vi "Ultrasonic Plot V2015.vi"(0 "Front L/R":cluster{i32, i32}, 4 "Limiter":i16=60, 5 "Y/X/Ang":cluster{"Y":i32, "X":i32, "Ring 2":T1} {"Ring 2" items=["0", "45", "90", "135", "180", "225", "270", "315"]}, 6 "error in (no error)":errorcluster, 7 "map reference in":refnum<data-value>) -> (1 "Runmap":bool, 2 "error out":errorcluster, 3 "map reference out":refnum<data-value>)   [LabVIEW 2014]
uses:
  <vilib>/robotics/Navigation/shared/WorldMap/OccupancyGridWorldMap/NI_Robotics_OccupancyGridWorldMap.lvclass
  Controls/Direction enum.ctl
panel:
  out "s? t:f":i32
  out "Angle":T1 items=["0", "45", "90", "135", "180", "225", "270", "315"]
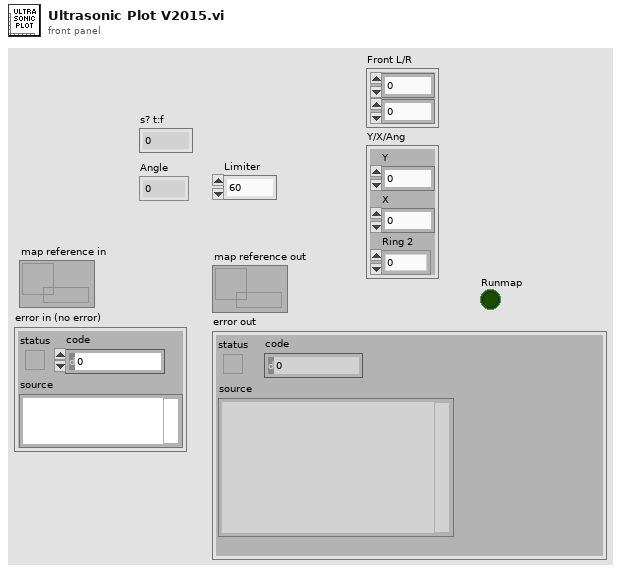
[diagram p1: front panel]
types:
  T1 = typedef "Direction enum.ctl" = u16
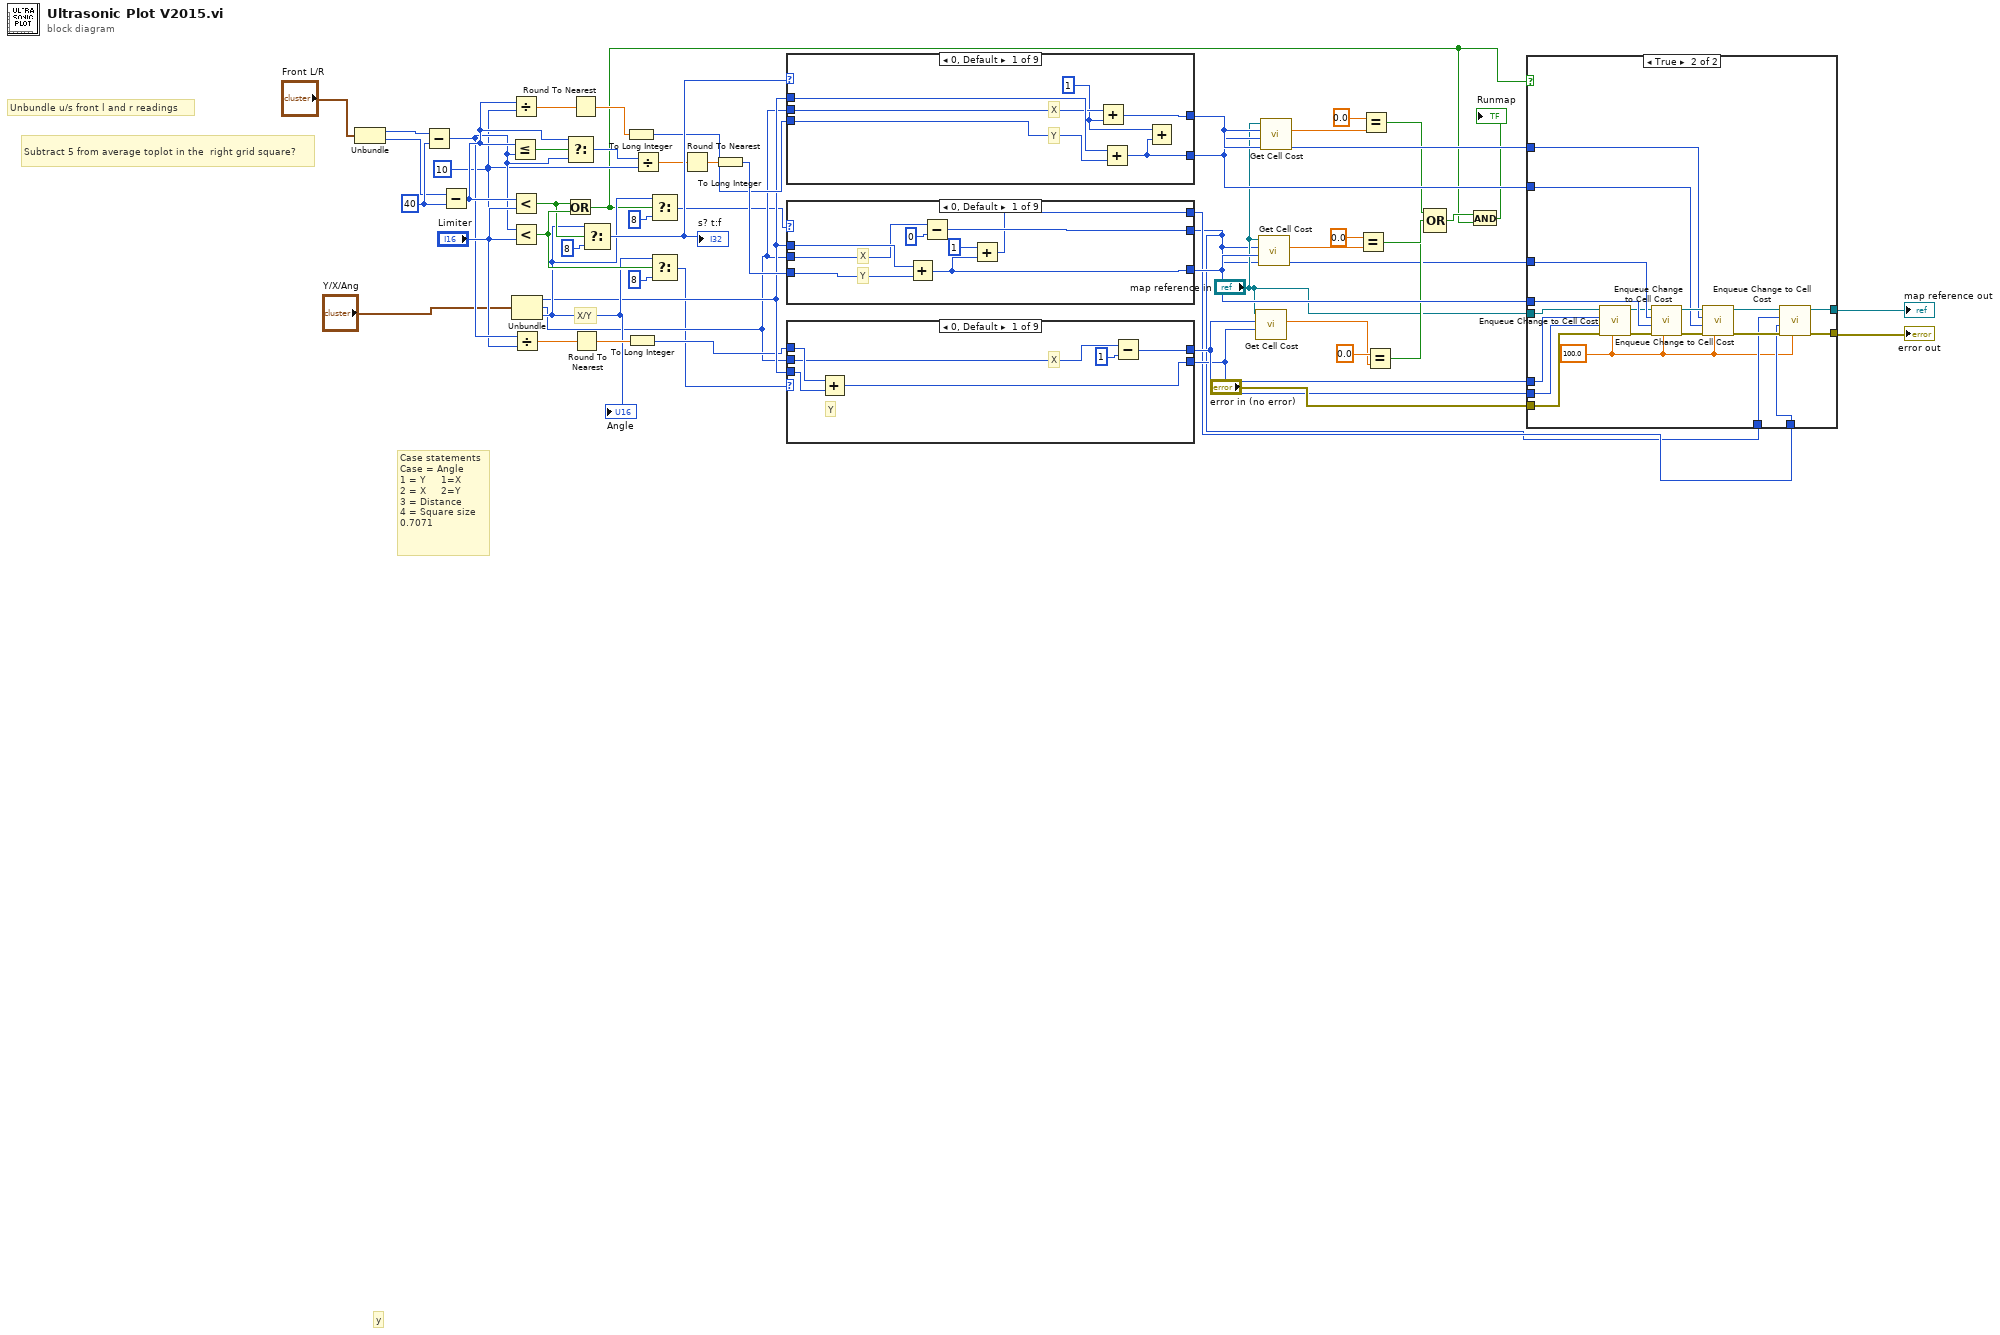
[diagram p0: block diagram]
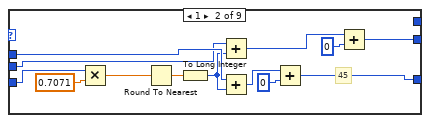
[diagram p2: hidden frame]
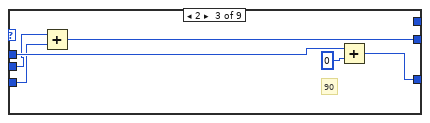
[diagram p3: hidden frame]
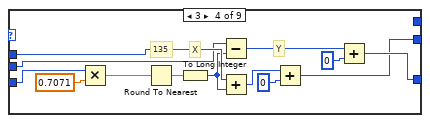
[diagram p4: hidden frame]
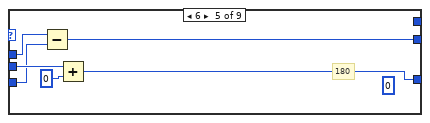
[diagram p5: hidden frame]
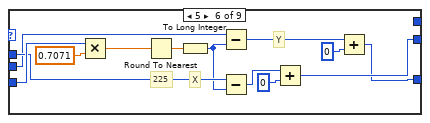
[diagram p6: hidden frame]
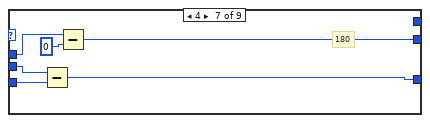
[diagram p7: hidden frame]
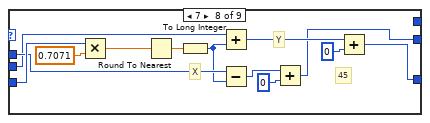
[diagram p8: hidden frame]
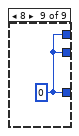
[diagram p9: hidden frame]
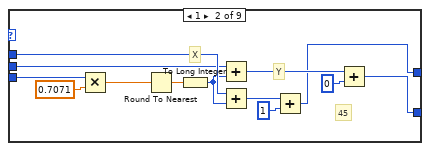
[diagram p10: hidden frame]
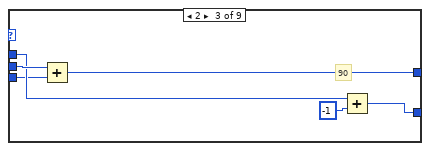
[diagram p11: hidden frame]
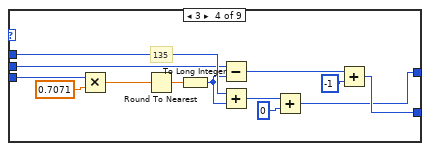
[diagram p12: hidden frame]
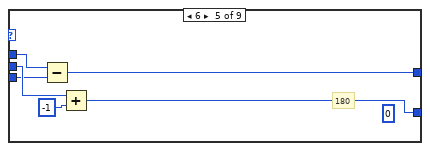
[diagram p13: hidden frame]
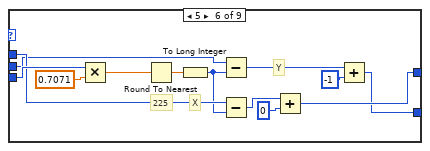
[diagram p14: hidden frame]
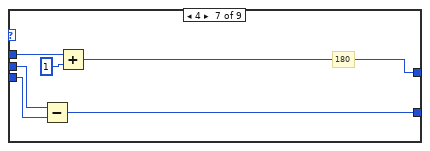
[diagram p15: hidden frame]
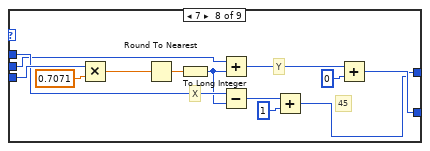
[diagram p16: hidden frame]
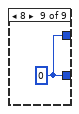
[diagram p17: hidden frame]
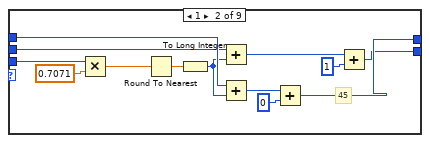
[diagram p18: hidden frame]
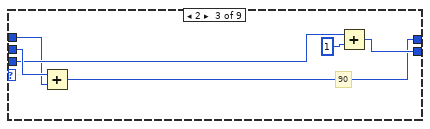
[diagram p19: hidden frame]
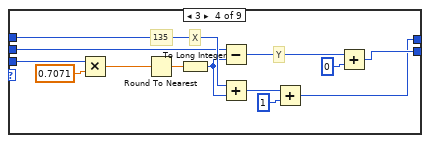
[diagram p20: hidden frame]
diagram:
  w37 = 40
  w33 = 10
  # "Subtract 5 from average toplot in the  right grid square?"
  # "Unbundle u/s front l and r readings"
  # "Case statements \nCase = Angle\n1 = Y     1=X\n2 = X     2=Y\n3 = Distance\n4 = Square size \n0.7071"
  # "y"
  # "X/Y"
  n1 = Unbundle("Front L/R") -> (w31:i32, w30:i32)
  n2 = Subtract(x=w31, y=w37) -> (x-y=w34:i32)
  n3 = Subtract(x=w30, y=w37) -> (x-y=w36:i32)
  n4 = Less Or Equal?(x=w36, y=w34) -> (x <= y?=w51:bool)
  n5 = Divide(x=w36, y=w33) -> (x/y=w45:dbl)
  n6 = Less?(x=w36, y="Limiter") -> (x < y?=w48:bool)
  n7 = Less?(x=w34, y="Limiter") -> (x < y?=w49:bool)
  n8 = Unbundle("Y/X/Ang") -> ("Y"=w7:i32, "X"=w5:i32, "Ring 2"=w27:T1)
  "Angle" <- w27
  n9 = Divide(x=w34, y=w33) -> (x/y=w35:dbl)
  n10 = Select(t=w36, s=w51, f=w34) -> (s? t:f=w42:i32)
  n11 = Or(x=w48, y=w49) -> (x .or. y?=w11:bool)
  n12 = Round To Nearest(number=w45) -> (nearest integer value=w46:dbl)
  n13 = Round To Nearest(number=w35) -> (nearest integer value=w32:dbl)
  n14 = Select(t=w27, s=w48, f=8) -> (s? t:f=w50:i32)
  "s? t:f" <- w50
  n15 = To Long Integer(number=w46) -> (32bit integer=w8:i32)
  n16 = To Long Integer(number=w32) -> (32bit integer=w6:i32)
  n17 = Divide(x=w42, y=w33) -> (x/y=w43:dbl)
  n18 = Select(t=w27, s=w11, f=8) -> (s? t:f=w4:i32)
  n19 = Select(t=w27, s=w49, f=8) -> (s? t:f=w1:i32)
  n20 = Round To Nearest(number=w43) -> (nearest integer value=w44:dbl)
  n21 = To Long Integer(number=w44) -> (32bit integer=w41:i32)
  n22 = case shown="0, Default" w50 {
    tunnel: w5 -> [w59 w68 w78 w87 w96 w106 w113 w125 _]
    tunnel: w7 -> [w60 w71 w77 w90 w97 w109 w116 w128 _]
    tunnel: w8 -> [w55 w73 w76 w92 w93 w111 w112 w130 _]
    tunnel: [w58 w61 w75 w80 w95 w100 w115 w118 w131] -> w26
    tunnel: [w56 w62 w74 w81 w94 w99 w114 w119 w131] -> w25
    frame 0, Default {
      w57 = 1
      # "Y"
      # "X"
      n23 = Add(x=w59, y=w57) -> (x+y=w58:i32)
      n24 = Add(x=w60, y=w55) -> (x+y=w56:i32)
      n25 = Add(x=w57, y=w56) -> ()  [unwired: 1 out]
    }
    frame 1 {
      # "Y"
      # "X"
      # "45"
      n26 = Multiply(x=w73, y=0.7071) -> (x*y=w63:dbl)
      n27 = Round To Nearest(number=w63) -> (nearest integer value=w69:dbl)
      n28 = To Long Integer(number=w69) -> (32bit integer=w67:i32)
      n29 = Add(x=w68, y=w67) -> (x+y=w64:i32)
      n30 = Add(x=w71, y=w67) -> (x+y=w65:i32)
      n31 = Add(x=w65, y=1) -> (x+y=w61:i32)
      n32 = Add(x=w64, y=0) -> (x+y=w62:i32)
    }
    frame 2 {
      # "90"
      n33 = Add(x=w78, y=w76) -> (x+y=w75:i32)
      n34 = Add(x=w77, y=-1) -> (x+y=w74:i32)
    }
    frame 3 {
      # "135"
      n35 = Multiply(x=w92, y=0.7071) -> (x*y=w82:dbl)
      n36 = Round To Nearest(number=w82) -> (nearest integer value=w88:dbl)
      n37 = To Long Integer(number=w88) -> (32bit integer=w86:i32)
      n38 = Subtract(x=w87, y=w86) -> (x-y=w83:i32)
      n39 = Add(x=w90, y=w86) -> (x+y=w84:i32)
      n40 = Add(x=w84, y=0) -> (x+y=w80:i32)
      n41 = Add(x=w83, y=-1) -> (x+y=w81:i32)
    }
    frame 6 {
      (unwired) 0
      # "180"
      n42 = Subtract(x=w97, y=w93) -> (x-y=w95:i32)
      n43 = Add(x=w96, y=-1) -> (x+y=w94:i32)
    }
    frame 5 {
      # "Y"
      # "X"
      # "225"
      n44 = Multiply(x=w111, y=0.7071) -> (x*y=w101:dbl)
      n45 = Round To Nearest(number=w101) -> (nearest integer value=w107:dbl)
      n46 = To Long Integer(number=w107) -> (32bit integer=w105:i32)
      n47 = Subtract(x=w106, y=w105) -> (x-y=w102:i32)
      n48 = Subtract(x=w109, y=w105) -> (x-y=w103:i32)
      n49 = Add(x=w103, y=0) -> (x+y=w100:i32)
      n50 = Add(x=w102, y=-1) -> (x+y=w99:i32)
    }
    frame 4 {
      # "180"
      n51 = Subtract(x=w113, y=w112) -> (x-y=w114:i32)
      n52 = Add(x=w116, y=1) -> (x+y=w115:i32)
    }
    frame 7 {
      # "Y"
      # "X"
      # "45"
      n53 = Multiply(x=w130, y=0.7071) -> (x*y=w120:dbl)
      n54 = Round To Nearest(number=w120) -> (nearest integer value=w126:dbl)
      n55 = To Long Integer(number=w126) -> (32bit integer=w124:i32)
      n56 = Add(x=w125, y=w124) -> (x+y=w121:i32)
      n57 = Subtract(x=w128, y=w124) -> (x-y=w122:i32)
      n58 = Add(x=w122, y=1) -> (x+y=w118:i32)
      n59 = Add(x=w121, y=0) -> (x+y=w119:i32)
    }
    frame 8 {
      w131 = 0
    }
  }
  n60 = case shown="0, Default" w4 {
    tunnel: w5 -> [w137 w146 w153 w166 w175 w185 w192 w204 _]
    tunnel: w7 -> [w138 w150 w157 w169 w176 w188 w195 w207 _]
    tunnel: w41 -> [w135 w152 w154 w171 w172 w190 w191 w209 _]
    tunnel: [w136 w147 w155 w159 w174 w179 w194 w197 w210] -> w2
    tunnel: [w134 w142 w156 w160 w173 w178 w193 w198 w210] -> w24
    tunnel: [w132 _ _ _ _ _ _ _ w210] -> w3
    frame 0, Default {
      # "Y"
      # "X"
      n61 = Add(x=w138, y=w135) -> (x+y=w134:i32)
      n62 = Subtract(x=w137, y=0) -> (x-y=w136:i32)
      n63 = Add(x=1, y=w134) -> (x+y=w132:i32)
    }
    frame 1 {
      # "45"
      n64 = Multiply(x=w152, y=0.7071) -> (x*y=w140:dbl)
      n65 = Round To Nearest(number=w140) -> (nearest integer value=w148:dbl)
      n66 = To Long Integer(number=w148) -> (32bit integer=w145:i32)
      n67 = Add(x=w146, y=w145) -> (x+y=w141:i32)
      n68 = Add(x=w150, y=w145) -> (x+y=w143:i32)
      n69 = Add(x=w143, y=0) -> (x+y=w142:i32)
      n70 = Add(x=w141, y=0) -> (x+y=w147:i32)
    }
    frame 2 {
      # "90"
      n71 = Add(x=w153, y=w154) -> (x+y=w155:i32)
      n72 = Add(x=w157, y=0) -> (x+y=w156:i32)
    }
    frame 3 {
      # "Y"
      # "X"
      # "135"
      n73 = Multiply(x=w171, y=0.7071) -> (x*y=w161:dbl)
      n74 = Round To Nearest(number=w161) -> (nearest integer value=w167:dbl)
      n75 = To Long Integer(number=w167) -> (32bit integer=w165:i32)
      n76 = Subtract(x=w166, y=w165) -> (x-y=w162:i32)
      n77 = Add(x=w169, y=w165) -> (x+y=w163:i32)
      n78 = Add(x=w163, y=0) -> (x+y=w159:i32)
      n79 = Add(x=w162, y=0) -> (x+y=w160:i32)
    }
    frame 6 {
      (unwired) 0
      # "180"
      n80 = Subtract(x=w176, y=w172) -> (x-y=w174:i32)
      n81 = Add(x=w175, y=0) -> (x+y=w173:i32)
    }
    frame 5 {
      # "Y"
      # "X"
      # "225"
      n82 = Multiply(x=w190, y=0.7071) -> (x*y=w180:dbl)
      n83 = Round To Nearest(number=w180) -> (nearest integer value=w186:dbl)
      n84 = To Long Integer(number=w186) -> (32bit integer=w184:i32)
      n85 = Subtract(x=w185, y=w184) -> (x-y=w181:i32)
      n86 = Subtract(x=w188, y=w184) -> (x-y=w182:i32)
      n87 = Add(x=w182, y=0) -> (x+y=w179:i32)
      n88 = Add(x=w181, y=0) -> (x+y=w178:i32)
    }
    frame 4 {
      # "180"
      n89 = Subtract(x=w192, y=w191) -> (x-y=w193:i32)
      n90 = Subtract(x=w195, y=0) -> (x-y=w194:i32)
    }
    frame 7 {
      # "Y"
      # "X"
      # "45"
      n91 = Multiply(x=w209, y=0.7071) -> (x*y=w199:dbl)
      n92 = Round To Nearest(number=w199) -> (nearest integer value=w205:dbl)
      n93 = To Long Integer(number=w205) -> (32bit integer=w203:i32)
      n94 = Add(x=w204, y=w203) -> (x+y=w200:i32)
      n95 = Subtract(x=w207, y=w203) -> (x-y=w201:i32)
      n96 = Add(x=w201, y=0) -> (x+y=w197:i32)
      n97 = Add(x=w200, y=0) -> (x+y=w198:i32)
    }
    frame 8 {
      w210 = 0
    }
  }
  n98 = case shown="0, Default" w1 {
    tunnel: w5 -> [w214 w224 w234 w243 w252 w262 w269 w281 _]
    tunnel: w6 -> [w215 w227 w232 w246 w253 w265 w272 w284 _]
    tunnel: w7 -> [w211 w229 w233 w248 w249 w267 w268 w286 _]
    tunnel: [w213 w218 w230 w236 w251 w255 w271 w274 w287] -> w23
    tunnel: [w212 w217 w231 w237 w250 w256 w270 w275 w287] -> w22
    frame 0, Default {
      # "Y"
      # "X"
      n99 = Add(x=w215, y=w211) -> (x+y=w212:i32)
      n100 = Subtract(x=w214, y=1) -> (x-y=w213:i32)
    }
    frame 1 {
      # "45"
      n101 = Multiply(x=w229, y=0.7071) -> (x*y=w219:dbl)
      n102 = Round To Nearest(number=w219) -> (nearest integer value=w225:dbl)
      n103 = To Long Integer(number=w225) -> (32bit integer=w223:i32)
      n104 = Add(x=w224, y=w223) -> (x+y=w220:i32)
      n105 = Add(x=w227, y=w223) -> (x+y=w221:i32)
      n106 = Add(x=w221, y=0) -> (x+y=w218:i32)
      n107 = Add(x=w220, y=1) -> (x+y=w217:i32)
    }
    frame 2 {
      # "90"
      n108 = Add(x=w234, y=w232) -> (x+y=w230:i32)
      n109 = Add(x=w233, y=1) -> (x+y=w231:i32)
    }
    frame 3 {
      # "Y"
      # "X"
      # "135"
      n110 = Multiply(x=w248, y=0.7071) -> (x*y=w238:dbl)
      n111 = Round To Nearest(number=w238) -> (nearest integer value=w244:dbl)
      n112 = To Long Integer(number=w244) -> (32bit integer=w242:i32)
      n113 = Subtract(x=w243, y=w242) -> (x-y=w239:i32)
      n114 = Add(x=w246, y=w242) -> (x+y=w240:i32)
      n115 = Add(x=w240, y=1) -> (x+y=w236:i32)
      n116 = Add(x=w239, y=0) -> (x+y=w237:i32)
    }
    frame 6 {
      (unwired) 0
      # "180"
      n117 = Subtract(x=w253, y=w249) -> (x-y=w251:i32)
      n118 = Add(x=w252, y=1) -> (x+y=w250:i32)
    }
    frame 5 {
      # "Y"
      # "X"
      # "225"
      n119 = Multiply(x=w267, y=0.7071) -> (x*y=w257:dbl)
      n120 = Round To Nearest(number=w257) -> (nearest integer value=w263:dbl)
      n121 = To Long Integer(number=w263) -> (32bit integer=w261:i32)
      n122 = Subtract(x=w262, y=w261) -> (x-y=w258:i32)
      n123 = Subtract(x=w265, y=w261) -> (x-y=w259:i32)
      n124 = Add(x=w259, y=-1) -> (x+y=w255:i32)
      n125 = Add(x=w258, y=0) -> (x+y=w256:i32)
    }
    frame 4 {
      # "180"
      n126 = Subtract(x=w269, y=w268) -> (x-y=w270:i32)
      n127 = Subtract(x=w272, y=1) -> (x-y=w271:i32)
    }
    frame 7 {
      # "Y"
      # "X"
      # "45"
      n128 = Multiply(x=w286, y=0.7071) -> (x*y=w276:dbl)
      n129 = Round To Nearest(number=w276) -> (nearest integer value=w282:dbl)
      n130 = To Long Integer(number=w282) -> (32bit integer=w280:i32)
      n131 = Add(x=w281, y=w280) -> (x+y=w277:i32)
      n132 = Subtract(x=w284, y=w280) -> (x-y=w278:i32)
      n133 = Add(x=w278, y=0) -> (x+y=w274:i32)
      n134 = Add(x=w277, y=-1) -> (x+y=w275:i32)
    }
    frame 8 {
      w287 = 0
    }
  }
  n135 = call <vilib>:"Get Cell Cost.vi"("y"=w22, "x"=w23, "map reference in"="map reference in") -> ("cost"=w16:dbl)  [unwired: 5 in, 3 out]
  n136 = call <vilib>:"Get Cell Cost.vi"("y"=w24, "x"=w2, "map reference in"="map reference in") -> ("cost"=w17:dbl)  [unwired: 5 in, 3 out]
  n137 = call <vilib>:"Get Cell Cost.vi"("y"=w25, "x"=w26, "map reference in"="map reference in") -> ("cost"=w18:dbl)  [unwired: 5 in, 3 out]
  n138 = Equal?(x=0.0, y=w17) -> (x = y?=w14:bool)
  n139 = Equal?(x=0.0, y=w18) -> (x = y?=w15:bool)
  n140 = Equal?(x=0.0, y=w16) -> (x = y?=w13:bool)
  n141 = Compound Arithmetic op=OR(w15, w14, w13) -> (w12:bool)
  n142 = And(x=w12, y=w11) -> (x .and. y?=→"Runmap":bool)
  n143 = case shown="True" w11 {
    tunnel: w24 -> [_ w308]
    tunnel: w2 -> [_ w307]
    tunnel: w22 -> [_ w306]
    tunnel: w23 -> [_ w305]
    tunnel: w26 -> [_ w297]
    tunnel: w25 -> [_ w302]
    tunnel: "map reference in" -> [w289 w299]
    tunnel: "error in (no error)" -> [w288 w298]
    tunnel: [w289 w296] -> w39
    tunnel: [w288 w295] -> w38
    tunnel: w2 -> [_ w292]
    tunnel: w3 -> [_ w291]
    frame False {
    }
    frame True {
      w290 = 100.0 ("cost")
      n144 = call <vilib>:"Enqueue Change to Cell Cost.vi"("cost"=w290, "error in (no error)"=w298, "y"=w306, "x"=w305, "map reference in"=w299) -> ("error out"=w300:errorcluster, "map reference out"=w301:refnum<data-value>)  [unwired: 5 in]
      n145 = call <vilib>:"Enqueue Change to Cell Cost.vi"("cost"=w290, "error in (no error)"=w300, "y"=w308, "x"=w307, "map reference in"=w301) -> ("error out"=w304:errorcluster, "map reference out"=w303:refnum<data-value>)  [unwired: 5 in]
      n146 = call <vilib>:"Enqueue Change to Cell Cost.vi"("cost"=w290, "error in (no error)"=w304, "y"=w302, "x"=w297, "map reference in"=w303) -> ("error out"=w293:errorcluster, "map reference out"=w294:refnum<data-value>)  [unwired: 5 in]
      n147 = call <vilib>:"Enqueue Change to Cell Cost.vi"("cost"=w290, "error in (no error)"=w293, "y"=w291, "x"=w292, "map reference in"=w294) -> ("error out"=w295:errorcluster, "map reference out"=w296:refnum<data-value>)  [unwired: 5 in]
    }
  }
  "map reference out" <- w39
  "error out" <- w38
